vi "Enable Key Lock.vi"(8 "error in (no error)":errorcluster, 10 "Enable Key Lock (F: False)":bool, 11 "VISA resource name":refnum<visa-resource-name>) -> (0 "error out":errorcluster, 3 "VISA resource name out":refnum<visa-resource-name>)   [LabVIEW 2015, in "BK Precision 983X Series.lvlib"]
doc: "Enables or disables key lock. When enabled, all keys in the front panel of the instrument are locked."
uses:
  <instrlib>/BK Precision 983X Series/BK Precision 983X Series.lvlib
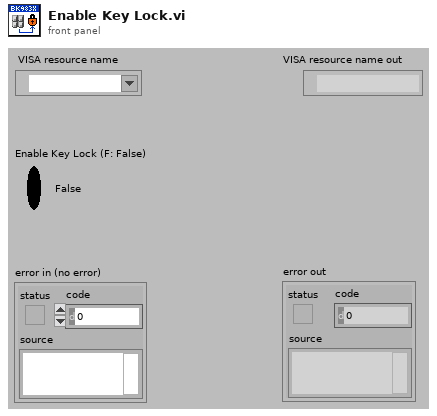
[diagram p1: front panel]
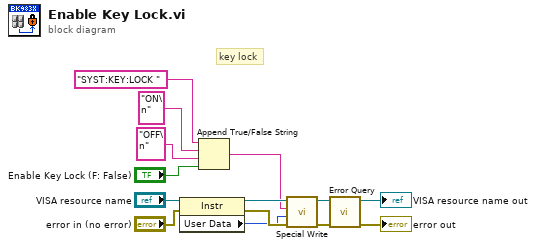
[diagram p0: block diagram]
diagram:
  # "key lock"
  n1 = property class="Instr"(reference="VISA resource name", error in="error in (no error)") -> (reference out=w4:refnum<visa-resource-name>, error out=w3:errorcluster, "User Data"=w2:u32)
  n2 = Append True/False String(1:"Enable Key Lock (F: False)", 2:"OFF\n" ("true string"), 3:"ON\n" ("true string"), 4:"SYST:KEY:LOCK ") -> (0:w1:string)
  n3 = call <instrlib>:"Special Write.vi"("error in (no error)"=w3, "Delay (0 ms)"=w2, "Input String"=w1, "VISA resource name"=w4) -> ("error out"=w7:errorcluster, "VISA resource name out"=w8:refnum<visa-resource-name>)  [unwired: 6 in]
  n4 = call <instrlib>:"Error Query.vi"("error in (no error)"=w7, "VISA resource name"=w8) -> ("error out"=→"error out":errorcluster, "VISA resource name out"=→"VISA resource name out":refnum<visa-resource-name>)  [unwired: 6 in, 2 out]
